vi "Get Current Time.vi"(8 "error in":errorcluster) -> (0 "error out":errorcluster, 3 "Current Time(s)":dbl format="%_19f")   [LabVIEW 2026, in "Template Engine.lvlib"]
uses:
  Template Engine.lvlib
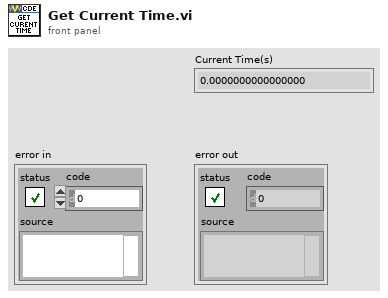
[diagram p1: front panel]
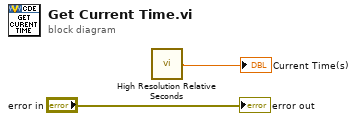
[diagram p0: block diagram]
diagram:
  n1 = call <vilib>:"High Resolution Relative Seconds.vi"() -> ("relative seconds"=→"Current Time(s)":dbl)
  "error out" <- "error in"
